vi "Auto-Indexing Tunels.vi"() -> ()   [LabVIEW 2020]
panel:
  out "Input Tunnel Result (Auto Index)":dbl
  out "Current Iteration":i32
  out "Output Tunnel Result":i32[](array[numeric])
  in  "1D DBL Array Input":dbl[](array[numeric])=[25.0, 50.0, 75.0, 100.0, 125.0, 150.0, 175.0, 200.0, 225.0, 250.0, 275.0, 300.0]
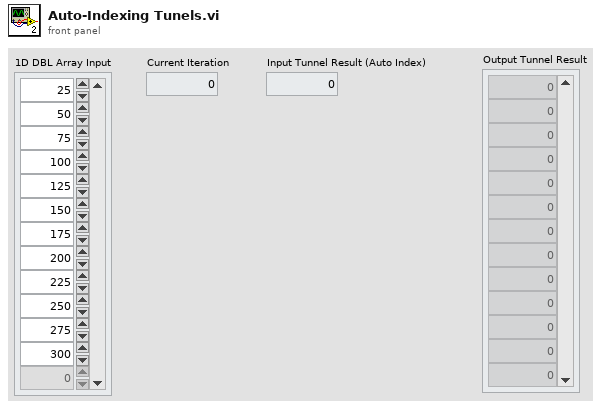
[diagram p1: front panel]
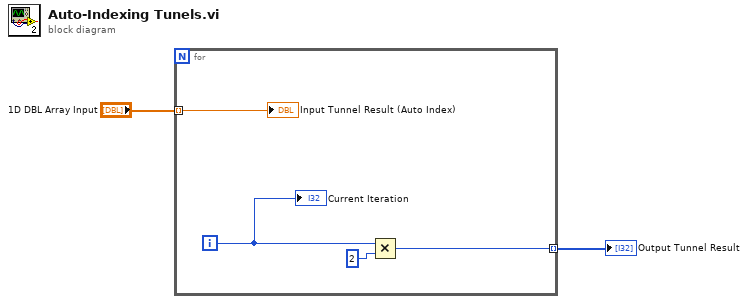
[diagram p0: block diagram]
diagram:
  n1 = for {
    tunnel: "1D DBL Array Input" -> [w4] mode=indexing
    tunnel: [w3] -> w1 mode=indexing
    i -> [w6]
    n2 = Multiply(x=w6, y=2) -> (x*y=w3:i32)
    "Input Tunnel Result (Auto Index)" <- w4
    "Current Iteration" <- w6
  }
  "Output Tunnel Result" <- w1
